vi "TB-Enqueue Mic Data.vi"(0 "state thru":T1, 9 "AI Waveforms in":dbl[][](array[numeric]), 11 "error in (no error)":errorcluster, 13 "Queue in":T4) -> (10 "AI Waveforms thru":dbl[][](array[numeric]), 15 "error out":errorcluster)   [LabVIEW 2020]
uses:
  Typedefs/TB-Mic Queue.ctl
  Typedefs/TB-Runtime state.ctl
  <vilib>/sound2/lvsound2.llb/Sound File Refnum.ctl
  Typedefs/TB-Setup Log.ctl
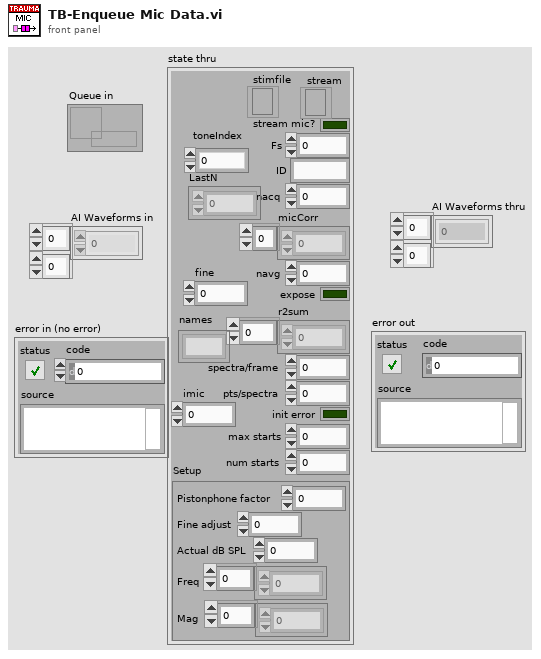
[diagram p1: front panel]
types:
  T1 = typedef "TB-Runtime state.ctl" = cluster{"stimfile":T2, "stream mic?":bool, "Fs":dbl, "ID":string, "micCorr":dbl[], "navg":i32, "r2sum":dbl[], "expose":bool, "spectra/frame":i32, "pts/spectra":i32, "nacq":i32, "init error":bool, "max starts":i32, "num starts":i32, "Setup":T3, "toneIndex":i32, "LastN":dbl[], "fine":dbl, "imic":i32, "stream":refnum<file>, "names":string[]}
  T2 = typedef "Sound File Refnum.ctl" = refnum<file>
  T3 = typedef "TB-Setup Log.ctl" = cluster{"Pistonphone factor":dbl, "Fine adjust":dbl, "Actual dB SPL":dbl, "Freq":dbl[], "Mag":dbl[]}
  T4 = typedef "TB-Mic Queue.ctl" = refnum<queue>
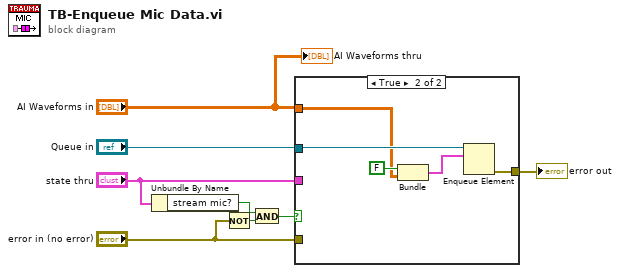
[diagram p0: block diagram]
diagram:
  n1 = Unbundle By Name("state thru") -> ("stream mic?"=w3:bool)
  n2 = Not(x="error in (no error)") -> (.not. x?=w5:bool)
  n3 = And(x=w3, y=w5) -> (x .and. y?=w6:bool)
  n4 = case shown="True" w6 {
    tunnel: [w9 w13] -> w7
    tunnel: "AI Waveforms in" -> [_ w10]
    tunnel: "state thru" -> [_ _]
    tunnel: "Queue in" -> [_ w14]
    tunnel: "error in (no error)" -> [w9 _]
    frame False {
    }
    frame True {
      n5 = Bundle(FALSE, "AI Waveforms in"=w10) -> (w11:cluster{bool, "AI Waveforms in":dbl[][]})  [unwired: 1 in]
      n6 = Enqueue Element(queue=w14, element=w11) -> (error out=w13:errorcluster)  [unwired: 2 in, 2 out]
    }
  }
  "error out" <- w7
  "AI Waveforms thru" <- "AI Waveforms in"
